vi "Configure Auto Mode Preset.vi"(8 "error in (no error)":errorcluster, 10 "preset index":u8(ring) items=["0", "1", "2", "3", "4", "5", "6", "7", "8", "9", "A", "B", "C"], 11 "MKS MW in":refnum<class "PL MKS MW.lvclass">) -> (0 "error out":errorcluster, 3 "MKS MW out":refnum<class "PL MKS MW.lvclass">)   [LabVIEW 2015, in "PL MKS MW.lvclass"]
doc: "Configure auto mode capacitor position <b>preset index</b>."
uses:
  PL MKS MW.lvclass
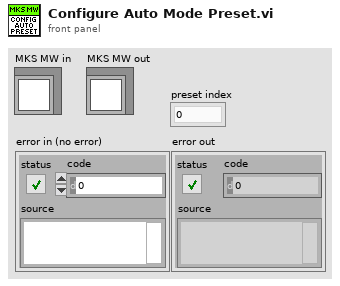
[diagram p1: front panel]
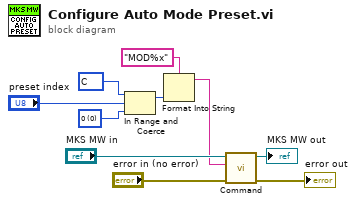
[diagram p0: block diagram]
diagram:
  w3 = u8 12 items=["0", "1", "2", "3", "4", "5", "6", "7", "8", "9", "A", "B", "C"] ("preset index")
  w2 = u8 0 items=["0", "1", "2", "3", "4", "5", "6", "7", "8", "9", "A", "B", "C"] ("preset index")
  n1 = In Range and Coerce(upper limit=w3, x="preset index", lower limit=w2) -> (coerced(x)=w5:u8)  [unwired: 1 out]
  n2 = Format Into String(format string="MOD%x", w5) -> (resulting string=w1:string)  [unwired: 2 in, 1 out]
  n3 = call "Command.vi"("error in (no error)"="error in (no error)", "command"=w1, "MKS MW in"="MKS MW in") -> ("error out"=→"error out":errorcluster, "MKS MW out"=→"MKS MW out":refnum<class "PL MKS MW.lvclass">)  [unwired: 6 in, 1 out]
